vi "Test.vi"() -> ()   [LabVIEW 2016]
uses:
  <vilib>/vision/driver/NI_Vision_Acquisition_Software.lvlib
  <vilib>/vision/NI_Vision_Development_Module.lvlib
panel:
  out "DeltaPos":cluster{dbl, dbl}[](array[cluster])
  out "Raw Pos":cluster{"x":sgl, "y":sgl}[](array[cluster])
  out "Pos wrt centre [pixels]":cluster{dbl, dbl}[](graph)
  out "Pos [pixels]":cluster{"x":sgl, "y":sgl}[](graph)
  in  "Pattern Match Settings":T1={"Algorithm"=2, "Number of Matches Requested"=1, "Minimum Match Score"=800.0, "SubPixel Accuracy"=TRUE, "Rotation Angle Ranges"=[], "Show Search Area"=FALSE, "Show Result"=TRUE} {"Rotation Angle Ranges"."End" format="%.1f"; "Rotation Angle Ranges"."Start" format="%.1f"; "Minimum Match Score" min=0 max=1000 format="%.2f"; "Number of Matches Requested" min=1; "Algorithm" items=["All", "Low Discrepancy Sampling", "Grayscale Value Pyramid", "Gradients Pyramid"]}
  out "File Data Type out":i32
  out "File Type out":string
  out "Template":T2(plugin-control)
  in  "Template File Path":path
  in  "OK Button - Dump":bool
  in  "Path to save collected images":path=path "C:/Users/Aerotech/Documents/Stave Assembly Records/2017-03-15/ATLAS07/FiducialsTestRun"
  in  "OK Button - Save":bool
  out "Error report":errorcluster
  in  "Camera Name":refnum<k21>="cam0" caption="IMAQdx Session"
  out "Most recently collected image":T2(plugin-control)
  out "Finished!":bool
  out "XYZ Stage Current Position":T3={"X [-750, 750 mm]"=-61.75289519379574, "Y [-150, 30 mm]"=-124.53559346701012, "Z [-50, 50 mm]"=-0.8115271662620002}
  in  "Axes Speeds [mm/s]":T4={"X Speed"=10.0, "Y Speed"=10.0, "Z Speed"=10.0}
  out "Moving":bool
  in  "Object Location [mm]":T5={"Go to X"=-61.753, "Go to Y"=-124.535, "Go to Z"=-0.811426}
  out "Image Array":T2[](array[plugin-control])
  out "Generated List of Coordinates":dbl[][](array[numeric])
  in  "A [mm]":cluster{"X":dbl, "Y":dbl, "Z":dbl}={"X"=-679.349, "Y"=-40.588, "Z"=-11.4218}
  # "Four Corner Check for Module"
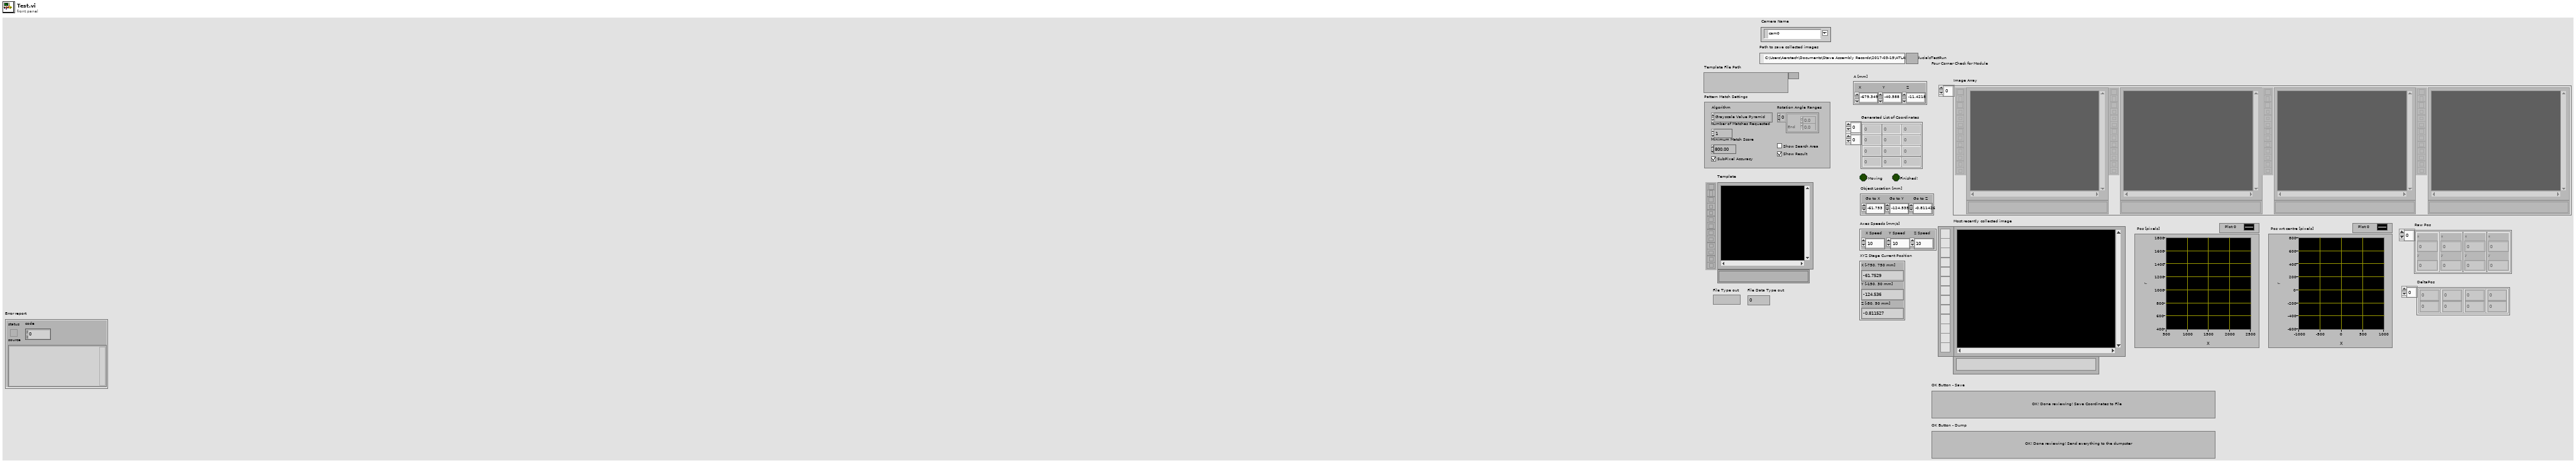
[diagram p1: front panel]
types:
  T1 = cluster{"Algorithm":i32, "Number of Matches Requested":i32, "Minimum Match Score":sgl, "SubPixel Accuracy":bool, "Rotation Angle Ranges":cluster{"Start":sgl, "End":sgl}[], "Show Search Area":bool, "Show Result":bool}
  T2 = typedef "IMAQ Image.ctl" = refnum<image>
  T3 = cluster{"X [-750, 750 mm]":dbl, "Y [-150, 30 mm]":dbl, "Z [-50, 50 mm]":dbl}
  T4 = cluster{"X Speed":dbl, "Y Speed":dbl, "Z Speed":dbl}
  T5 = cluster{"Go to X":dbl, "Go to Y":dbl, "Go to Z":dbl}
  T6 = typedef "IMAQdx.ctl" = refnum<k21>
  T7 = cluster{"Generated List of Coordinates[0]":dbl, "Generated List of Coordinates[1]":dbl, "Generated List of Coordinates[2]":dbl}
  T8 = typedef "Image Type" = u32
  T9 = cluster{"Final X":dbl, "Final Y":dbl, "Final Z":dbl}
  T10 = cluster{"Position":cluster{"x":sgl, "y":sgl}, "Angle":sgl, "Scale":sgl, "Score":sgl, "Bounding Box":cluster{"x":sgl, "y":sgl}[]}[]
  T11 = cluster{"Position":cluster{"x":sgl, "y":sgl}, "Angle":sgl, "Scale":sgl, "Score":sgl, "Bounding Box":cluster{"x":sgl, "y":sgl}[]}
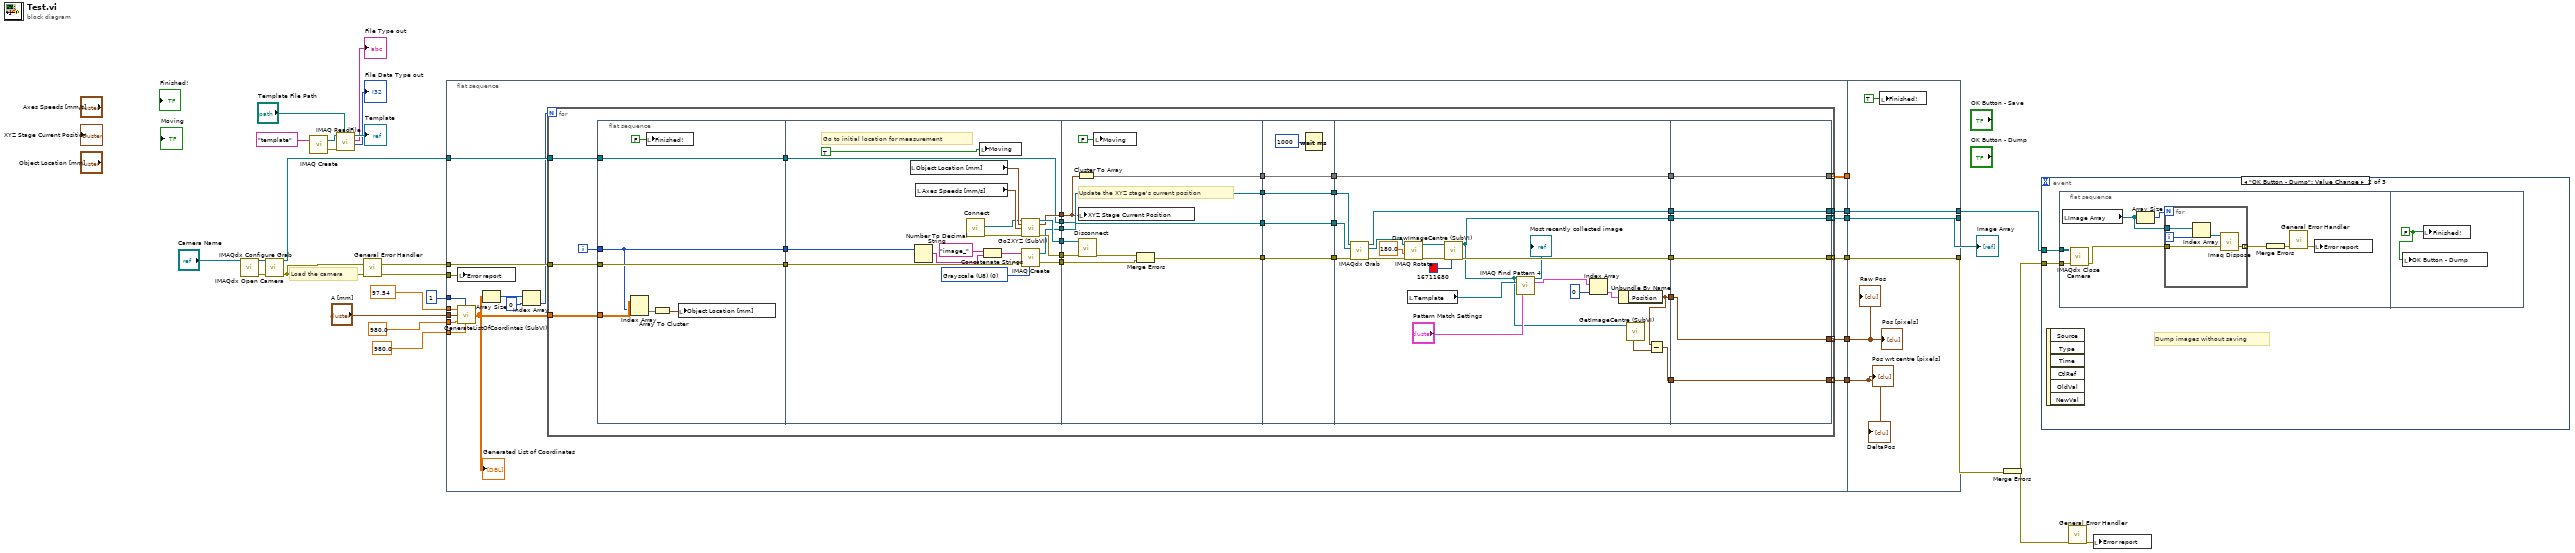
[diagram p0: block diagram]
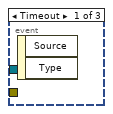
[diagram p2: hidden frame]
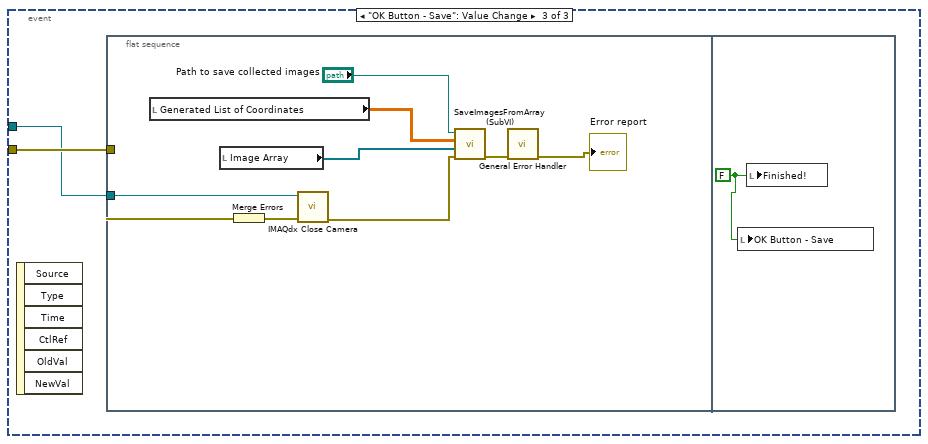
[diagram p3: hidden frame]
diagram:
  # "Load the camera"
  n1 = call <vilib>:"IMAQdx Open Camera.vi"("Session In"="Camera Name") -> ("error out"=w23:errorcluster, "Session Out"=w24:T6)  [unwired: 2 in, 7 out]
  n2 = call <vilib>:"IMAQdx Configure Grab.vi"("error in"=w23, "Session In"=w24) -> ("error out"=w20:errorcluster, "Session Out"=w19:T6)  [unwired: 8 out]
  n3 = call "IMAQ Create"("Image Name"="template") -> ("New Image"=w8:T2, "error out"=w9:errorcluster)  [unwired: 4 in]
  n4 = call "IMAQ ReadFile"("File Path"="Template File Path", "error in (no error)"=w9, "Image"=w8) -> ("File Data Type out"=→"File Data Type out":i32, "File Type out"=→"File Type out":string, "Image Out"=→"Template":T2)  [unwired: 4 in, 2 out]
  n5 = call <vilib>:"General Error Handler.vi"("error in (no error)"=w20) -> ("error out"=w21:errorcluster)  [unwired: 2 in, 12 out]
  n6 = flat-sequence {
    tunnel: 97.54 ("Module side length [mm]") -> [w47]
    tunnel: "A [mm]" -> [w46]
    tunnel: 980.0 ("x to fiducial [um]") -> [w45]
    tunnel: 980.0 ("y to fiducial [um]") -> [w44]
    tunnel: 1 ("Nloops") -> [w43]
    tunnel: w21 -> [w42]
    tunnel: w20 -> [w41]
    tunnel: w19 -> [w40]
    tunnel: [w39] -> w16
    tunnel: [w38] -> w15
    tunnel: [w37] -> w13
    tunnel: [w36] -> w11
    tunnel: [w31] -> w2
    tunnel: [w30] -> w1
    tunnel: w16 -> [w152]
    tunnel: [w152] -> w14
    tunnel: w15 -> [_]
    tunnel: w13 -> [w150]
    tunnel: [w150] -> w12
    tunnel: w11 -> [w151]
    tunnel: [w151] -> w10
    tunnel: w2 -> [w149]
    tunnel: w1 -> [w148]
    frame #0 {
      n7 = local write "Error report"(w42) -> ()
      n8 = call "GenerateListOfCoordintes (SubVI).vi"("Module side length [mm]"=w47, "Nloops"=w43, "A [mm]"=w46, "x to fiducial [um]"=w45, "y to fiducial [um]"=w44) -> ("Generated List of Coordinates"=w35:dbl[][])  [unwired: 4 in]
      "Generated List of Coordinates" <- w35
      n9 = Array Size(array=w35) -> (size(s)=w34:i32[])
      n10 = Index Array(array=w34, index=0) -> (element=w33:i32)
      n11 = for {
        N: w33 -> [_]
        tunnel: w35 -> [w64]
        tunnel: w41 -> [w63]
        tunnel: w40 -> [w62]
        tunnel: [w60] -> w39 mode=indexing
        tunnel: [w59] -> w38 mode=indexing
        tunnel: [w58] -> w37 mode=indexing
        tunnel: [w57] -> w36
        tunnel: [w50] -> w31 mode=indexing
        tunnel: [w48] -> w30 mode=indexing
        i -> [w61]
        n12 = flat-sequence {
          tunnel: [w85] -> w80
          tunnel: w62 -> [w85]
          tunnel: [w84] -> w79
          tunnel: w63 -> [w84]
          tunnel: w64 -> [w82]
          tunnel: w61 -> [w81]
          tunnel: [w81] -> w56
          tunnel: [w98] -> w78
          tunnel: [w97] -> w77
          tunnel: [w96] -> w76
          tunnel: [w93] -> w75
          tunnel: [w92] -> w74
          tunnel: w80 -> [w92]
          tunnel: w79 -> [w90]
          tunnel: [w89] -> w73
          tunnel: w56 -> [w88]
          tunnel: w78 -> [w113]
          tunnel: w77 -> [w106]
          tunnel: w76 -> [w112]
          tunnel: [w111] -> w72
          tunnel: w75 -> [w111]
          tunnel: [w110] -> w71
          tunnel: w74 -> [w110]
          tunnel: [w107] -> w70
          tunnel: w73 -> [w108]
          tunnel: [w105] -> w69
          tunnel: [w118] -> w68
          tunnel: w72 -> [w118]
          tunnel: [w117] -> w67
          tunnel: w71 -> [w117]
          tunnel: [w116] -> w66
          tunnel: w70 -> [w116]
          tunnel: w69 -> [w115]
          tunnel: [w115] -> w65
          tunnel: w68 -> [w141]
          tunnel: w67 -> [w140]
          tunnel: w66 -> [w137]
          tunnel: w65 -> [w134]
          tunnel: [w123] -> w55
          tunnel: [w135] -> w54
          tunnel: [w131] -> w53
          tunnel: [w134] -> w52
          tunnel: [w121] -> w51
          tunnel: [w120] -> w49
          tunnel: [w144] -> w59
          tunnel: [w145] -> w58
          tunnel: [w146] -> w57
          tunnel: [w147] -> w60
          tunnel: w55 -> [w147]
          tunnel: w54 -> [w146]
          tunnel: w53 -> [w145]
          tunnel: w52 -> [w144]
          tunnel: w51 -> [w143]
          tunnel: [w143] -> w50
          tunnel: [w142] -> w48
          tunnel: w49 -> [w142]
          frame #0 {
            n13 = Index Array(array=w82, index (row)=w81) -> (element=w86:dbl[])  [unwired: 1 in]
            n14 = local write "Finished!"(FALSE ("Finished!")) -> ()
            n15 = Array To Cluster(array=w86) -> (cluster=w87:T7)
            n16 = local write "Object Location [mm]"(w87) -> ()
          }
          frame #1 {
            w104 = T8 0 items=["Grayscale (U8)", "Grayscale (I16)", "Grayscale (SGL)", "Complex (CSG)", "RGB (U32)", "HSL (U32)", "RGB (U64)", "Grayscale (U16)"] ("Image Type")
            # "Go to initial location for measurement"
            n17 = local read "Object Location [mm]"() -> (w101:T5)
            n18 = Number To Decimal String(number=w88) -> (decimal integer string=w91:string)  [unwired: 1 in]
            n19 = local read "Axes Speeds [mm/s]"() -> (w102:T4)
            n20 = call "Connect.vi"() -> ("error out"=w99:errorcluster, "controller"=w100:refnum<k24>)  [unwired: 10 in]
            n21 = local write "Moving"(TRUE ("Moving")) -> ()
            n22 = Concatenate Strings("image_" ("Image Name"), w91) -> (w94:string)
            n23 = call "Go2XYZ (SubVI).vi"(".NET Refnum in"=w100, "Go to Coordinates"=w101, "Axis Speeds"=w102, "error in (no error)"=w99) -> (".NET Refnum out"=w98:refnum<k24>, "Final Position"=w97:T9, "error out"=w96:errorcluster)  [unwired: 8 in, 1 out]
            n24 = call "IMAQ Create"("Image Name"=w94, "Image Type"=w104, "error in (no error)"=w90) -> ("New Image"=w93:T2, "error out"=w89:errorcluster)  [unwired: 1 in, 1 out]
          }
          frame #2 {
            # "Update the XYZ stage's current position"
            n25 = Cluster To Array(cluster=w106) -> (array=w105:dbl[])
            n26 = local write "XYZ Stage Current Position"(w106) -> ()
            n27 = call "Disconnect.vi"("error in (no error)"=w112, "controller"=w113) -> ("error out"=w109:errorcluster)  [unwired: 9 in]
            n28 = local write "Moving"(FALSE ("Moving")) -> ()
            n29 = Merge Errors(w109, w108) -> (w107:errorcluster)
          }
          frame #3 {
            n30 = Wait (ms)(milliseconds to wait=u32 1000) -> ()  [unwired: 1 out]
          }
          frame #4 {
            n31 = call <vilib>:"IMAQdx Grab.vi"("error in"=w137, "Image In"=w141, "Session In"=w140) -> ("error out"=w136:errorcluster, "Image Out"=w139:T2, "Session Out"=w135:T6)  [unwired: 1 in, 5 out]
            n32 = call "IMAQ Rotate"("error in (no error)"=w136, "Angle (degrees)"=sgl 180.0, "Image Src"=w139) -> ("error out"=w132:errorcluster, "Image Dst Out"=w133:T2)  [unwired: 7 in]
            n33 = local read "Template"() -> (w129:T2)
            n34 = call "DrawImageCentre (SubVI).vi"("Axis colour"=u32 16711680, "error in (no error)"=w132, "Refnum in"=w133) -> ("error out"=w131:errorcluster, "Refnum out"=w123:T2)  [unwired: 7 in]
            n35 = call "IMAQ Find Pattern 4"("Image"=w123, "Template"=w129, "Settings"="Pattern Match Settings") -> ("Image Out"=→"Most recently collected image":T2, "Matches (pixel)"=w126:T10)  [unwired: 6 in, 5 out]
            n36 = Index Array(array=w126, index=0) -> (element=w124:T11)
            n37 = Unbundle By Name(w124) -> ("Position"=w121:cluster{"x":sgl, "y":sgl})
            n38 = call "GetImageCentre (SubVI).vi"("Image in \n(refnum)"=w123) -> ("Centre Point"=w122:cluster{"X coordinate":dbl, "Y coordinate":dbl})  [unwired: 4 in, 4 out]
            n39 = Subtract(x=w121, y=w122) -> (x-y=w120:cluster{dbl, dbl})
          }
          frame #5 {
          }
        }
      }
    }
    frame #1 {
      n40 = local write "Finished!"(TRUE ("Finished!")) -> ()
      "Pos [pixels]" <- w149
      "Pos wrt centre [pixels]" <- w148
      "Raw Pos" <- w149
      "DeltaPos" <- w148
    }
  }
  n41 = Merge Errors(w12) -> (w17:errorcluster)
  n42 = event shown="[1] \"OK Button - Dump\": Value Change" {
    selector: _ -> [_ _ _]
    dyn-events: _ -> [_ _ _]
    timeout: _ -> [_ _ _]
    tunnel: w17 -> [_ w155 w171]
    tunnel: w10 -> [_ w154 w170]
    event Timeout {
      n43 = event-data() -> ()  [unwired: 1 in, 2 out]
    }
    event "OK Button - Dump": Value Change {
      # "Dump images without saving"
      n44 = event-data() -> ()  [unwired: 1 in, 6 out]
      n45 = flat-sequence {
        tunnel: w155 -> [w163]
        tunnel: w154 -> [w156]
        frame #0 {
          n46 = local read "Image Array"() -> (w162:T2[])
          n47 = call <vilib>:"IMAQdx Close Camera.vi"("error in"=w163, "Session In"=w156) -> ("error out"=w159:errorcluster)  [unwired: 9 out]
          n48 = Array Size(array=w162) -> (size(s)=w161:i32)
          n49 = for {
            N: w161 -> [_]
            tunnel: w162 -> [w168]
            tunnel: w159 -> [w165]
            tunnel: [w164] -> w158 mode=indexing
            i -> [w167]
            n50 = Index Array(array=w168, index=w167) -> (element=w166:T2)
            n51 = call "Imaq Dispose"("Image"=w166, "error in (no error)"=w165) -> ("error out"=w164:errorcluster)  [unwired: 4 in]
          }
          n52 = Merge Errors(w158) -> (w157:errorcluster)
          n53 = call <vilib>:"General Error Handler.vi"("error in (no error)"=w157) -> ("error out"=w160:errorcluster)  [unwired: 2 in, 12 out]
          n54 = local write "Error report"(w160) -> ()
        }
        frame #1 {
          w169 = FALSE ("Finished!")
          n55 = local write "OK Button - Dump"(w169) -> ()
          n56 = local write "Finished!"(w169) -> ()
        }
      }
    }
    event "OK Button - Save": Value Change {
      n57 = event-data() -> ()  [unwired: 1 in, 6 out]
      n58 = flat-sequence {
        tunnel: w171 -> [w179]
        tunnel: w170 -> [w172]
        frame #0 {
          n59 = local read "Generated List of Coordinates"() -> (w174:dbl[][])
          n60 = local read "Image Array"() -> (w178:T2[])
          n61 = Merge Errors(w179) -> (w180:errorcluster)
          n62 = call <vilib>:"IMAQdx Close Camera.vi"("error in"=w180, "Session In"=w172) -> ("error out"=w177:errorcluster)  [unwired: 9 out]
          n63 = call "SaveImagesFromArray (SubVI).vi"("error in (no error)"=w177, "Array of Images"=w178, "XY Camera Coordinates"=w174, "Path to save collected images"="Path to save collected images") -> ("error out"=w176:errorcluster)  [unwired: 7 in]
          n64 = call <vilib>:"General Error Handler.vi"("error in (no error)"=w176) -> ("error out"=→"Error report":errorcluster)  [unwired: 2 in, 12 out]
        }
        frame #1 {
          w181 = FALSE ("Finished!")
          n65 = local write "OK Button - Save"(w181) -> ()
          n66 = local write "Finished!"(w181) -> ()
        }
      }
    }
  }
  n67 = call <vilib>:"General Error Handler.vi"("error in (no error)"=w17) -> ("error out"=w18:errorcluster)  [unwired: 2 in, 12 out]
  n68 = local write "Error report"(w18) -> ()
  "Image Array" <- w14
